vi "DROPBEAR_Model_Updating_FFT_KF.vi"(8 "error in (no error)":errorcluster, 11 "DROPBEAR_Model_Updating in":refnum<class "DROPBEAR_Model_Updating.lvclass">) -> (0 "error out":errorcluster, 3 "DROPBEAR_Model_Updating out":refnum<class "DROPBEAR_Model_Updating.lvclass">)   [LabVIEW 2021, in "DROPBEAR_Model_Updating.lvclass"]
uses:
  DROPBEAR_Model_Updating.lvclass
  DROPBEAR_Model_Updating.lvclass/DROPBEAR_Model_Updating.ctl
  Kalman_Filter/Kalman_Filter.lvclass
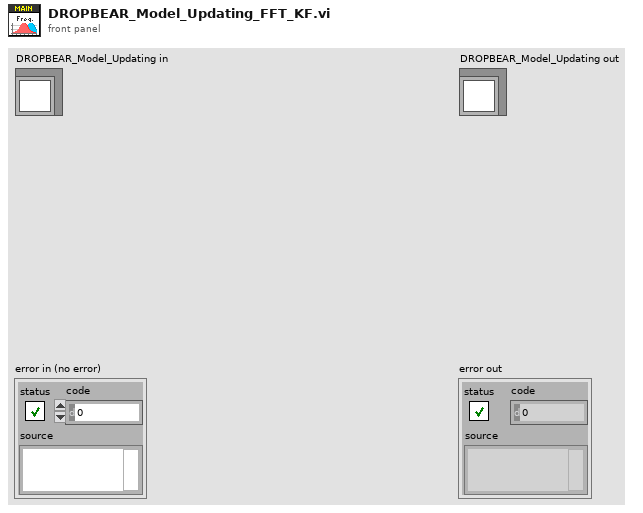
[diagram p1: front panel]
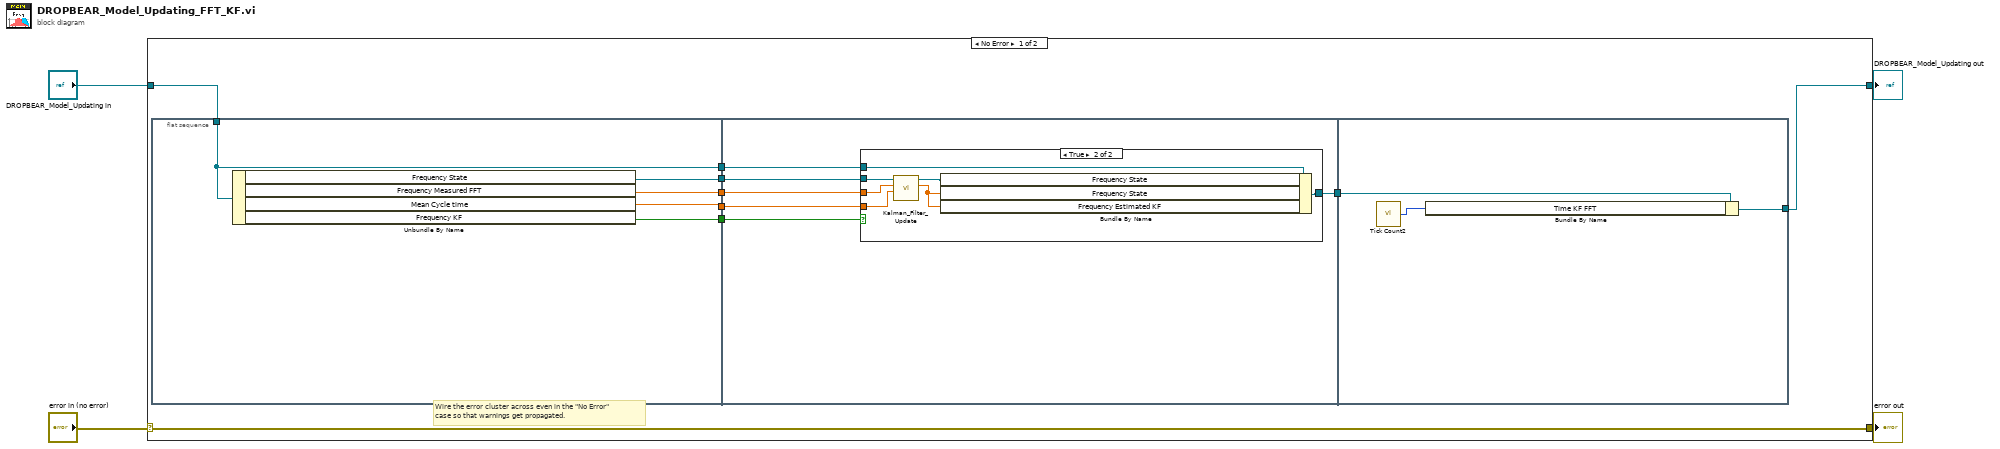
[diagram p0: block diagram]
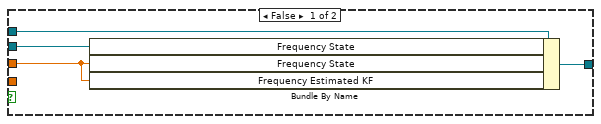
[diagram p2: hidden frame]
diagram:
  n1 = case shown="No Error" "error in (no error)" {
    selector: "error in (no error)" -> [w13 w40]
    tunnel: [w13 w40] -> w3
    tunnel: [w5 w39] -> w1
    tunnel: "DROPBEAR_Model_Updating in" -> [w12 w39]
    frame No Error {
      # "Wire the error cluster across even in the \"No Error\"\ncase so that warnings get propagated."
      n2 = flat-sequence {
        tunnel: w12 -> [w15]
        tunnel: [w18] -> w11
        tunnel: [w17] -> w10
        tunnel: [w16] -> w9
        tunnel: [w15] -> w8
        tunnel: [w14] -> w7
        tunnel: w11 -> [w24]
        tunnel: w10 -> [w23]
        tunnel: w9 -> [w22]
        tunnel: w8 -> [w21]
        tunnel: w7 -> [w20]
        tunnel: [w19] -> w6
        tunnel: w6 -> [w38]
        tunnel: [w37] -> w5
        frame #0 {
          n3 = Unbundle By Name(w15) -> ("Frequency State"=w18:refnum<class "Kalman_Filter.lvclass">, "Frequency Measured FFT"=w17:dbl, "Mean Cycle time"=w16:dbl, "Frequency KF"=w14:bool)
        }
        frame #1 {
          n4 = case shown="True" w20 {
            tunnel: w24 -> [w25 w33]
            tunnel: w23 -> [w26 w35]
            tunnel: w22 -> [_ w34]
            tunnel: w21 -> [w27 w32]
            tunnel: [w28 w30] -> w19
            frame False {
              n5 = Bundle By Name(cluster=w27, "Frequency State"=w25, "Frequency State"=w26, "Frequency Estimated KF"=w26) -> (w28:refnum<class "DROPBEAR_Model_Updating.lvclass">)
            }
            frame True {
              n6 = call "Kalman_Filter_Update.vi"("T Sample"=w34, "New Measurement"=w35, "Kalman_Filter in"=w33) -> ("Estimate"=w29:dbl, "Kalman_Filter out"=w31:refnum<class "Kalman_Filter.lvclass">)  [unwired: 6 in, 1 out]
              n7 = Bundle By Name(cluster=w32, "Frequency State"=w31, "Frequency State"=w29, "Frequency Estimated KF"=w29) -> (w30:refnum<class "DROPBEAR_Model_Updating.lvclass">)
            }
          }
        }
        frame #2 {
          n8 = call "Tick Count2"() -> ("Tick Count(uSec)"=w36:u32)
          n9 = Bundle By Name(cluster=w38, "Time KF FFT"=w36) -> (w37:refnum<class "DROPBEAR_Model_Updating.lvclass">)
        }
      }
    }
    frame Error {
    }
  }
  "error out" <- w3
  "DROPBEAR_Model_Updating out" <- w1
